vi "VescRead.vi"() -> (2 "RPM Out":dbl, 3 "Raw Out":string)   [LabVIEW 2019]
uses:
  <vilib>/myRIO/Instrument Drivers/Onboard IO/UART/typedef/VISA Configuration.ctl
  <vilib>/Instr/_visa.llb/VISA Configure Serial Port (Instr).vi
  <vilib>/myRIO/Express VI/Onboard IO/UART/UART Express VI.xnode
  <vilib>/myRIO/Instrument Drivers/Onboard IO/UART/UART.lvlib
  usr/local/lib/libvescEncoder.so
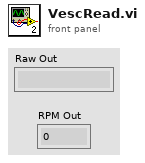
[diagram p1: front panel]
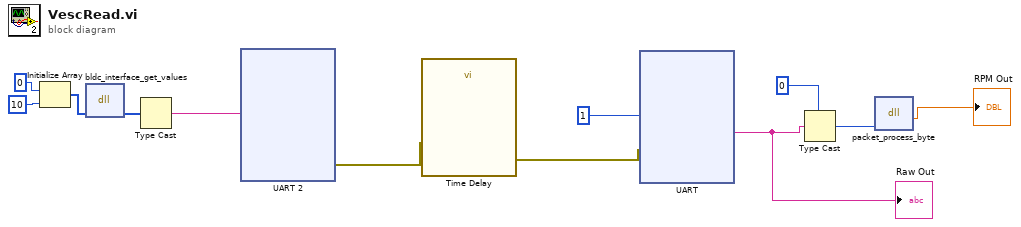
[diagram p0: block diagram]
diagram:
  n1 = Initialize Array(0, 10) -> (w6:i32[])
  n2 = dll-call lib="usr/local/lib/libvescEncoder.so" fn="bldc_interface_get_values"("array"=w6) -> ("array"=w5:u8[])  [unwired: 4 in, 2 out]
  n3 = Type Cast(x=w5) -> (*(type *) &x=w9:string)  [unwired: 1 in]
  n4 = xnode "UART 2"("Characters to Write"=w9) -> ("error out"=w4:errorcluster)  [unwired: 1 in, 1 out]
  n5 = call "Time Delay"("error in (no error)"=w4) -> ("error out"=w3:errorcluster)  [unwired: 10 in]
  n6 = xnode "UART"("Character Count"=1, "error in (no error)"=w3) -> ("Characters Read"=w2:string)  [unwired: 1 out]
  "Raw Out" <- w2
  n7 = Type Cast(type=u8 0, x=w2) -> (*(type *) &x=w12:u8)
  n8 = dll-call lib="usr/local/lib/libvescEncoder.so" fn="packet_process_byte"("rx_data"=w12) -> ("return type"=→"RPM Out":sgl)  [unwired: 4 in, 2 out]
